vi "InitNI-DAQ_Class.vi"(0 "DAQmx Device Name":tag, 1 "Physical channels":string[](array[string]), 5 "Number of channels":i32, 7 "Ranges and couplings":T1 {"Input terminal configuration" items=["default"=-1, "RSE"=10083, "NRSE"=10078, "Differential"=10106, "Pseudodifferential"=12529]}, 9 "Clock and trigger":T3={"Sample clock source"="None", "Sample mode"=10123, "Sample clock rate"=1000.0, "Samples per channel"=1000, "Trigger type"=enum."Immediate", "Trigger source"="None", "Pretrigger samples"=0} {"Sample clock rate" format="%#_6p"; "Sample mode" items=["Finite Samples"=10178, "Continuous Samples"=10123, "Hardware Timed Single Point"=12522]}, 11 "error in (no error)":errorcluster, 12 "buffer size (in samples per channel)":u32) -> (4 "task out":refnum<k21>, 15 "error out":errorcluster)   [LabVIEW 2015]
uses:
  Controls/Ranges and coupling.ctl
  Controls/Range and coupling.ctl
  <vilib>/DAQmx/create/channels.llb/DAQmx Create Channel (AI-Voltage-Basic).vi
  <vilib>/DAQmx/configure/timing.llb/DAQmx Timing (Sample Clock).vi
  <vilib>/DAQmx/configure/trigger.llb/DAQmx Reference Trigger (Digital Edge).vi
  <vilib>/DAQmx/configure/trigger.llb/DAQmx Start Trigger (None).vi
  <vilib>/DAQmx/configure/trigger.llb/DAQmx Start Trigger (Digital Edge).vi
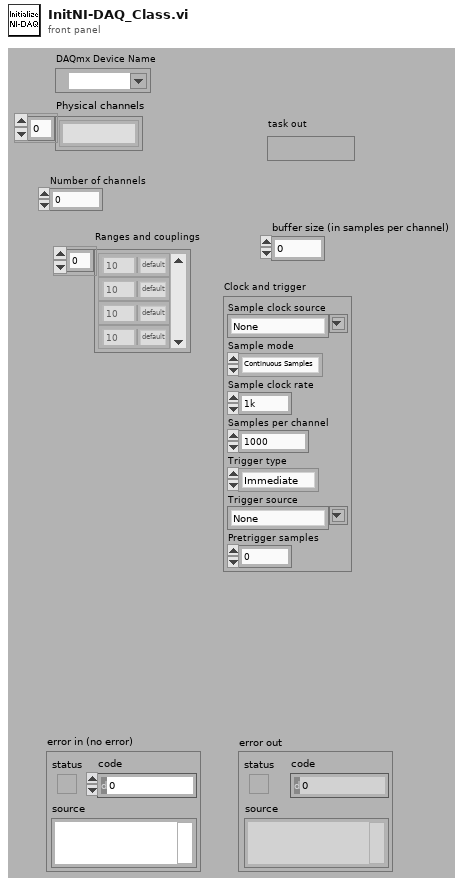
[diagram p1: front panel]
types:
  T1 = typedef "Ranges and coupling.ctl" = T2[]
  T2 = typedef "Range and coupling.ctl" = cluster{"Range":dbl, "Input terminal configuration":i32}
  T3 = cluster{"Sample clock source":string, "Sample mode":i32, "Sample clock rate":dbl, "Samples per channel":i32, "Trigger type":enum16{"Reference", "Immediate", "Start"}, "Trigger source":string, "Pretrigger samples":u32}
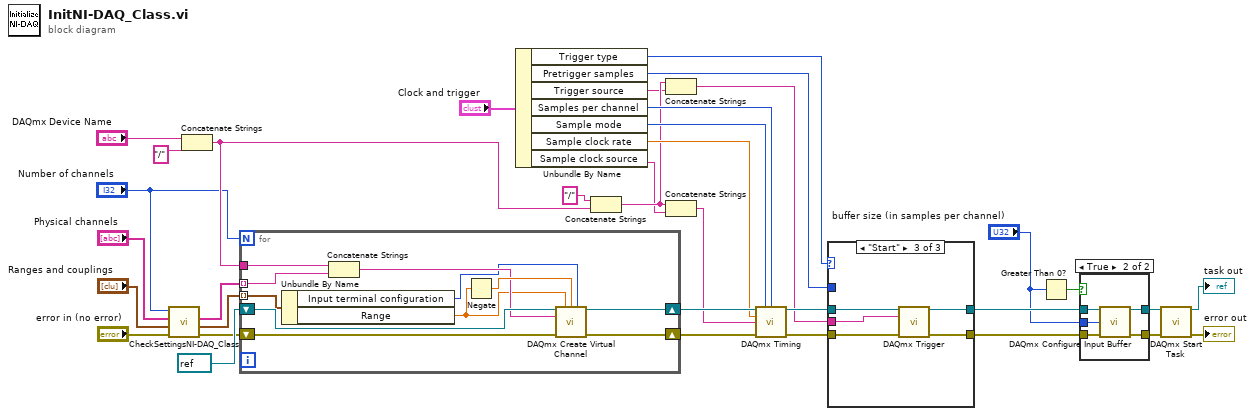
[diagram p0: block diagram]
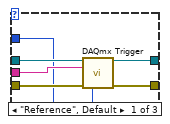
[diagram p3: hidden frame]
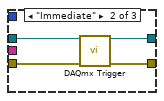
[diagram p4: hidden frame]
diagram:
  n1 = call "CheckSettingsNI-DAQ_Class.vi"("error in (no error)"="error in (no error)", "Ranges and couplings"="Ranges and couplings", "Physical channels"="Physical channels", "Number of channels"="Number of channels") -> ("error out"=w29:errorcluster, "Ranges and couplings  out"=w9:T1, "Physical channels out"=w16:string[])  [unwired: 5 in]
  n2 = Concatenate Strings("DAQmx Device Name", "/" ("string")) -> (w28:string)
  n3 = for {
    N: "Number of channels" -> [_]
    shift-right: [w46] -> w33
    shift-left: refnum<k21> refnum ("No task") -> [w42]
    shift-right: [w45] -> w32
    shift-left: w29 -> [w44]
    tunnel: w16 -> [w41] mode=indexing
    tunnel: w28 -> [w40]
    tunnel: w9 -> [w38] mode=indexing
    n4 = Unbundle By Name(w38) -> ("Input terminal configuration"=w36:i32, "Range"=w37:dbl)
    n5 = Concatenate Strings(w40, w41) -> (w39:string)
    n6 = Negate(x=w37) -> (-x=w43:dbl)
    n7 = call-poly <vilib>:"DAQmx Create Virtual Channel.vi"("task in"=w42, "maximum value"=w37, "minimum value"=w43, "input terminal configuration"=w36, "physical channels"=w39, "error in"=w44) -> ("task out"=w46:refnum<k21>, "error out"=w45:errorcluster)  [unwired: 3 in, 5 out]
  }
  n8 = Unbundle By Name("Clock and trigger") -> ("Trigger type"=w19:enum16{"Reference", "Immediate", "Start"}, "Pretrigger samples"=w11:u32, "Trigger source"=w12:string, "Samples per channel"=w23:i32, "Sample mode"=w24:i32, "Sample clock rate"=w22:dbl, "Sample clock source"=w1:string)
  n9 = Concatenate Strings("/" ("string"), w28) -> (w18:string)
  n10 = Concatenate Strings(w18, w12) -> (w25:string)
  n11 = Concatenate Strings(w18, w1) -> (w26:string)
  n12 = call-poly <vilib>:"DAQmx Timing.vi"("task/channels in"=w33, "sample mode"=w24, "samples per channel"=w23, "rate"=w22, "source"=w26, "error in"=w32) -> ("task out"=w34:refnum<k21>, "error out"=w35:errorcluster)  [unwired: 1 in, 7 out]
  n13 = case shown="\"Start\"" w19 {
    tunnel: w35 -> [w52 w56 w61]
    tunnel: w34 -> [w51 w55 w60]
    tunnel: w25 -> [w50 _ w59]
    tunnel: [w49 w54 w58] -> w6
    tunnel: [w48 w53 w57] -> w8
    tunnel: w11 -> [w47 _ _]
    frame "Reference", Default {
      n14 = call-poly <vilib>:"DAQmx Trigger.vi"("task/channels in"=w51, "source"=w50, "error in"=w52, "pretrigger samples per channel"=w47) -> ("task out"=w48:refnum<k21>, "error out"=w49:errorcluster)  [unwired: 1 in, 9 out]
    }
    frame "Immediate" {
      n15 = call-poly <vilib>:"DAQmx Trigger.vi"("task/channels in"=w55, "error in"=w56) -> ("task out"=w53:refnum<k21>, "error out"=w54:errorcluster)  [unwired: 3 in, 9 out]
    }
    frame "Start" {
      n16 = call-poly <vilib>:"DAQmx Trigger.vi"("task/channels in"=w60, "source"=w59, "error in"=w61) -> ("task out"=w57:refnum<k21>, "error out"=w58:errorcluster)  [unwired: 2 in, 9 out]
    }
  }
  n17 = Greater Than 0?(x="buffer size (in samples per channel)") -> (x > 0?=w4:bool)
  n18 = case shown="True" w4 {
    tunnel: w8 -> [w62 w68]
    tunnel: [w62 w67] -> w7
    tunnel: w6 -> [w63 w66]
    tunnel: [w63 w65] -> w5
    tunnel: "buffer size (in samples per channel)" -> [_ w64]
    frame False {
    }
    frame True {
      n19 = call <vilib>:"DAQmx Configure Input Buffer.vi"("task/channels in"=w68, "buffer size (in samples per channel)"=w64, "error in"=w66) -> ("task out"=w67:refnum<k21>, "error out"=w65:errorcluster)  [unwired: 11 in]
    }
  }
  n20 = call <vilib>:"DAQmx Start Task.vi"("task/channels in"=w7, "error in"=w5) -> ("task out"=→"task out":refnum<k21>, "error out"=→"error out":errorcluster)  [unwired: 12 out]
